vi "2D&3D Plots & Waweforms.vi"() -> ()   [LabVIEW 2014]
uses:
  <vilib>/LVH/AR Drone Toolkit/Decode NavData/Typedefs/NavData Demo.ctl
  <vilib>/Native 3D Graph/xcontrol/3DPC_SurfacePlot.xctl
  <vilib>/Native 3D Graph/classes/Line/Line.lvclass
  <vilib>/LVH/AR Drone Toolkit/AR Drone.lvlib
panel:
  out "Battery Remaining":dbl(slide)=97.0 scale=0.0..100.0
  out "vx":sgl(graph)
  out "vy":sgl(graph)
  out "Altitude":u32(graph)
  out "Tilt":T1(graph)={"pitch (deg)"=0.068, "roll (deg)"=-0.016, "yaw (deg)"=0.828}
  out "3D Graph":refnum<class "Base Datatype.lvclass">[](xcontrol)
  out "NavData Out":T2={"control state"=enum."TRANS_LANDING", "battery percentage"=97, "pitch (deg)"=0.068, "roll (deg)"=-0.016, "yaw (deg)"=0.828, "altitude (cm)"=0, "vx (cm/s)?"=0.0, "vy (cm/s)?"=0.0, "vz (cm/s)?"=0.0, "detection cam type"=3}
  out "nav":errorcluster
  out "ctr":errorcluster
  out "XY Graph":cluster{"Y":dbl[], "Y":dbl[]}[](graph)
  in  "stop":bool
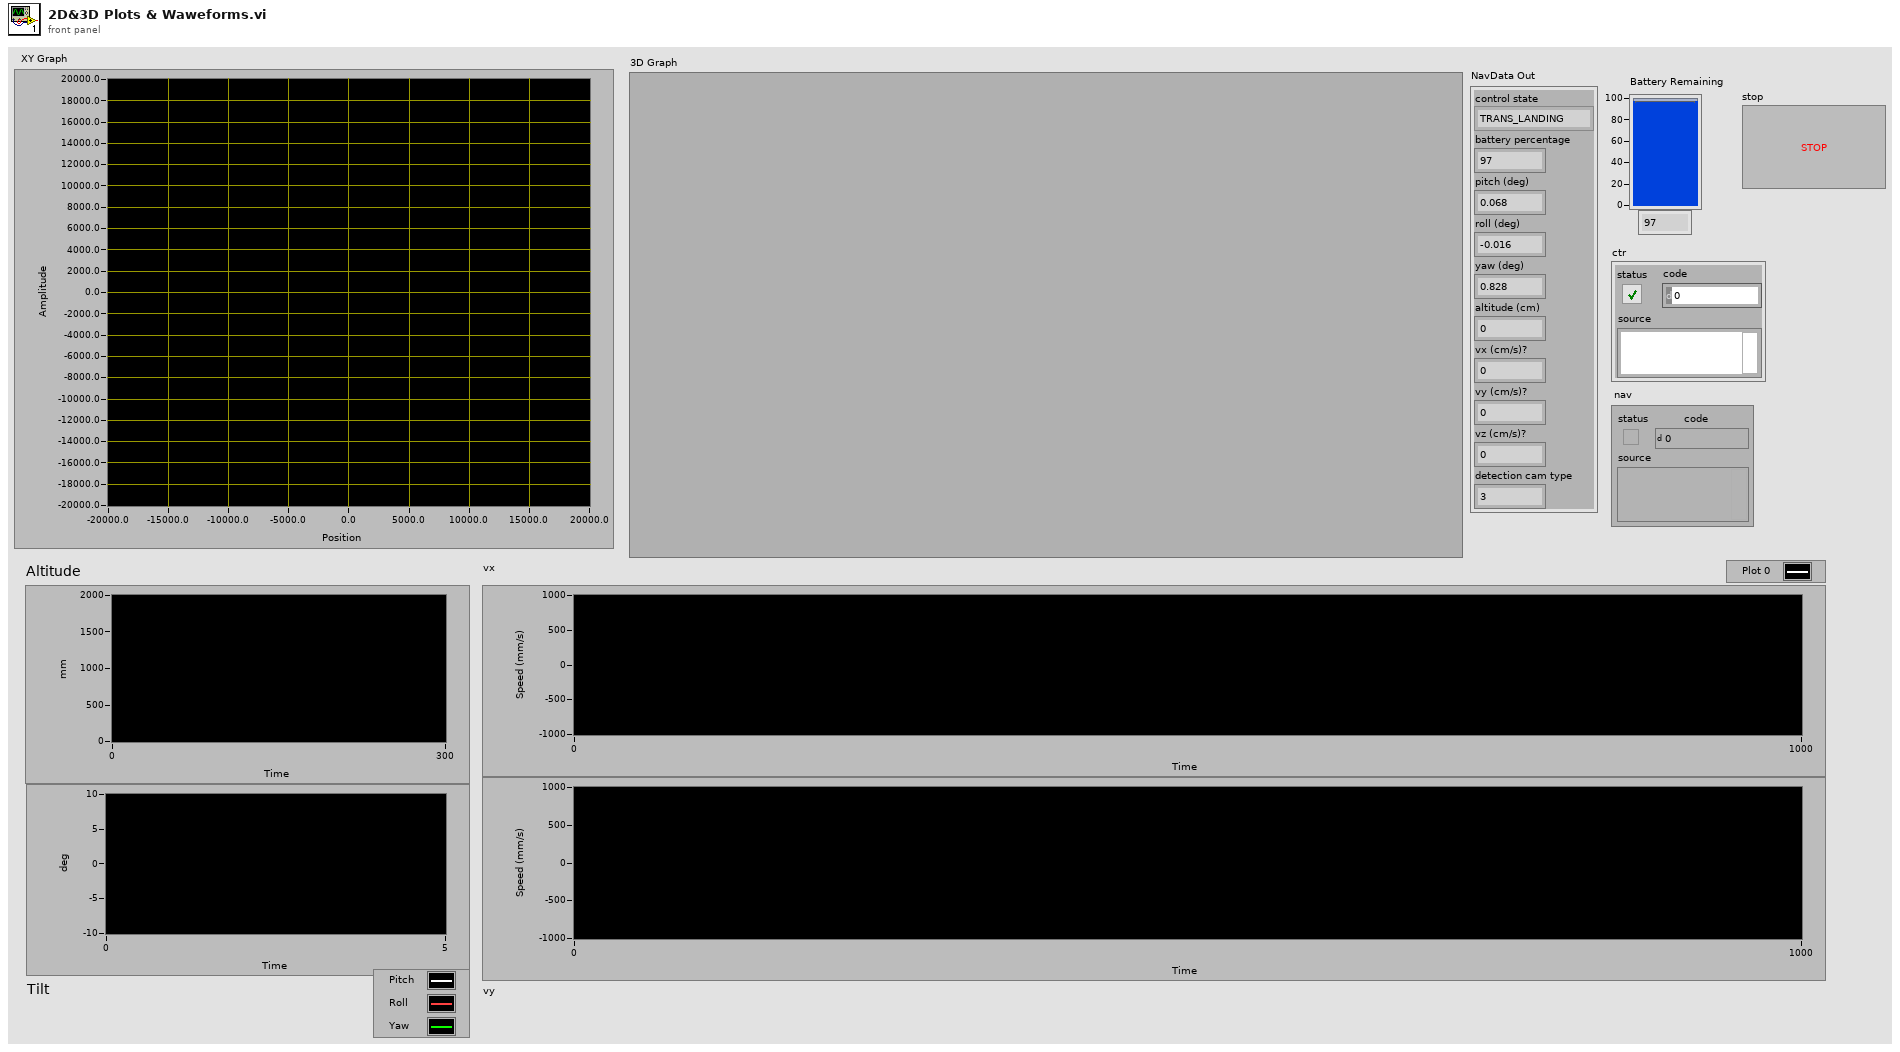
[diagram p1: front panel]
types:
  T1 = cluster{"pitch (deg)":sgl, "roll (deg)":sgl, "yaw (deg)":sgl}
  T2 = typedef "AR Drone.lvlib/NavData Demo.ctl" = cluster{"control state":enum32{"DEFAULT", "INIT", "LANDING", "FLYING", "HOVERING", "TEST", "TRANS_TAKEOFF", "TRANS_GOTOFIX", "TRANS_LANDING"}, "battery percentage":u32, "pitch (deg)":sgl, "roll (deg)":sgl, "yaw (deg)":sgl, "altitude (cm)":u32, "vx (cm/s)?":sgl, "vy (cm/s)?":sgl, "vz (cm/s)?":sgl, "detection cam type":u32}
  T3 = typedef "AR Drone.lvlib/AR Drone Resource.ctl" = cluster{"UDP Control Connection":refnum<k16>, "UDP NavData Connection":refnum<k16>, "UDP Video Connection (Drone 1.0)":refnum<k16>, "TCP Video Connection (Drone 2.0)":refnum<k5>, "TCP Control Port Connection":refnum<k5>, "Drone IP address":string, "Drone Command Port":u16, "Drone NavData Port":u16, "Drone Vid Stream Port":u16, "Drone TCP Control Port":u16, "Home IP address":string, "Home Command Port":u16, "Home NavData Port":u16, "Home Vid Stream Port":u16, "Drone Version":i32, "Drone Index":i32, "Command Sequence":i32}
  T4 = cluster{"Hover":bool, "Land/Take off":bool, "button 3":bool, "button 4":bool}
  T5 = cluster{"Roll":dbl, "Pitch":dbl, "Vertical Speed":dbl, "Yaw Speed":dbl}
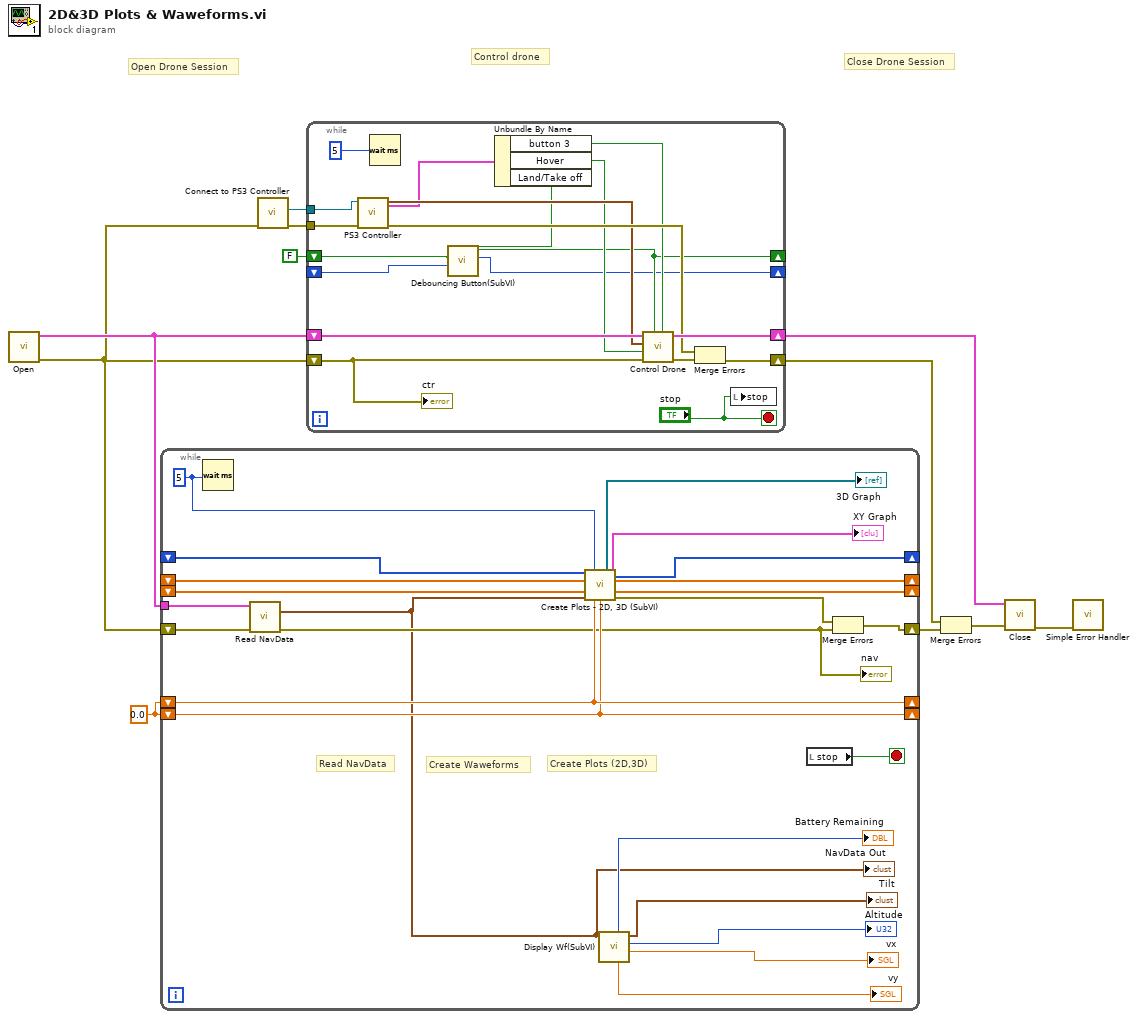
[diagram p0: block diagram]
diagram:
  w5 = 0.0
  # "Control drone"
  # "Close Drone Session"
  # "Open Drone Session"
  n1 = call <vilib>:"Open.vi"() -> ("error out"=w1:errorcluster, "AR Drone Resource"=w2:T3)  [unwired: 10 in]
  n2 = while {
    shift-right: [w13] -> w8
    shift-left: w1 -> [w32]
    shift-right: [w29] -> _
    shift-left: _ -> [w20]
    shift-right: [w28] -> _
    shift-left: _ -> [w31]
    shift-right: [w17] -> _
    shift-left: w5 -> [w17]
    shift-right: [w18] -> _
    shift-left: w5 -> [w18]
    shift-right: [w26] -> _
    shift-left: _ -> [w27]
    tunnel: w2 -> [w33]
    stop <- w34 stop-if-true
    w19 = u32 5 ("milliseconds to wait")
    # "Create Waweforms"
    # "Create Plots (2D,3D)"
    # "Read NavData"
    n3 = Wait (ms)(milliseconds to wait=w19) -> ()  [unwired: 1 out]
    n4 = call <vilib>:"Read NavData.vi"("error in (no error)"=w32, "AR Drone Resource"=w33) -> ("error out"=w15:errorcluster, "NavData Out"=w12:T2)  [unwired: 7 in, 1 out]
    "nav" <- w15
    "NavData Out" <- w12
    n5 = call "Create Plots - 2D, 3D (SubVI).vi"("Array in"=w27, "milliseconds to wait"=w19, "X array in"=w20, "Y array in"=w31, "NavData Out"=w12, "Numeric 2"=w18, "Numeric"=w17) -> ("3D Graph"=→"3D Graph":refnum<class "Base Datatype.lvclass">[], "XY Graph"=→"XY Graph":cluster{"Y":dbl[], "Y":dbl[]}[], "Array out"=w26:u32[], "X array out"=w29:dbl[], "Y array out"=w28:dbl[], "error out"=w16:errorcluster)  [unwired: 3 in]
    n6 = call "Display Wf(SubVI).vi"("NavData Out"=w12) -> ("vx (cm/s)?"=→"vx":sgl, "altitude (cm)"=→"Altitude":u32, "Cluster"=→"Tilt":T1, "vy (cm/s)?"=→"vy":sgl, "battery percentage"=→"Battery Remaining":u32)  [unwired: 6 in]
    n7 = local read "stop"() -> (w34:bool)
    n8 = Merge Errors(w16, w15) -> (w13:errorcluster)
  }
  n9 = call "Connect to PS3 Controller.vi"("error in (no error)"=w1) -> ("error out"=w7:errorcluster, "device ID 2"=w6:refnum<k1>)  [unwired: 8 in]
  n10 = while {
    shift-right: [w52] -> w11
    shift-left: w2 -> [w53]
    shift-right: [w47] -> w9
    shift-left: w1 -> [w46]
    tunnel: w7 -> [w50]
    tunnel: w6 -> [w35]
    shift-right: [w39] -> _
    shift-left: FALSE ("Boolean out") -> [w41]
    shift-right: [w38] -> _
    shift-left: _ -> [w37]
    stop <- "stop" stop-if-true
    n11 = call "PS3 Controller.vi"("error in (no error)"=w50, "device ID"=w35) -> ("error out"=w48:errorcluster, "Buttons control"=w44:T4, "Control cluster"=w45:T5)  [unwired: 7 in]
    n12 = Wait (ms)(milliseconds to wait=u32 5) -> ()  [unwired: 1 out]
    n13 = Unbundle By Name(w44) -> ("button 3"=w42:bool, "Hover"=w43:bool, "Land/Take off"=w40:bool)
    n14 = call "Debouncing Button(SubVI).vi"("millisecond timer value in"=w37, "Boolean in"=w41, "Land/Take off"=w40) -> ("millisecond timer value out"=w38:u32, "Boolean out"=w39:bool)  [unwired: 7 in]
    n15 = call <vilib>:"Control Drone.vi"("Emergency Landing"=w42, "Takeoff/Land"=w39, "error in (no error)"=w46, "Hover"=w43, "Control Cluster"=w45, "AR Drone Resource"=w53) -> ("error out"=w49:errorcluster, "AR Drone Resource Out"=w52:T3)  [unwired: 4 in]
    n16 = Merge Errors(w48, w49) -> (w47:errorcluster)
    n17 = local write "stop"("stop") -> ()
    "ctr" <- w46
  }
  n18 = Merge Errors(w9, w8) -> (w3:errorcluster)
  n19 = call <vilib>:"Close.vi"("error in (no error)"=w3, "AR Drone Resource"=w11) -> ("error out"=w10:errorcluster)  [unwired: 9 in]
  n20 = call <vilib>:"Simple Error Handler.vi"("error in (no error)"=w10) -> ()  [unwired: 4 in, 5 out]
